vi "Positions Should Turn.vi"(8 "column":i32, 9 "row":i32, 10 "chess color":T2=1, 11 "chesses":T1=[[0, 1, 2, 0, 0, 0, 0], [0, 2, 1, 0, 0, 0, 0], [0, 0, 0, 2, 0, 0, 0], [0, 0, 0, 0, 0, 0, 0], [0, 0, 0, 0, 0, 0, 0]]) -> (1 "positons to turn":i32[][](array[numeric]), 3 "chesses new":T1=[[0, 1, 2, 0, 0, 0, 0], [0, 2, 1, 0, 0, 0, 0], [0, 0, 0, 2, 0, 0, 0], [0, 0, 0, 0, 0, 0, 0], [0, 0, 0, 0, 0, 0, 0]])   [LabVIEW 2018, in "Othello.xctl"]
doc: "本VI是为《我和LabVIEW》一书编写的示例。\n关于本书的介绍请参考网页：\nhttp://ruanqizhen.spaces.live.com/blog/cns!5852D4F797C53FB6!4310.entry"
uses:
  Othello.xctl
  Control/Pict Ring Chess.ctl
  Ability/Data.ctl
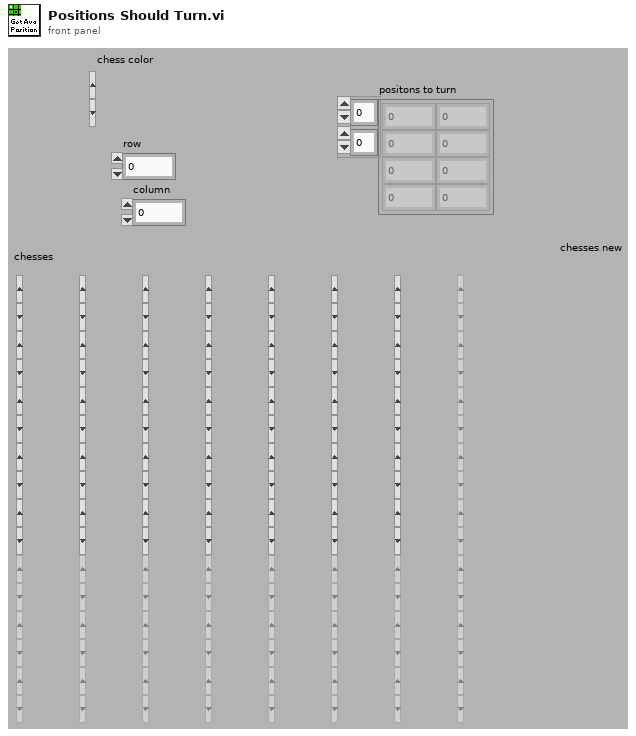
[diagram p1: front panel]
types:
  T1 = typedef "Othello.xctl/Data.ctl" = T2[][]
  T2 = typedef "Othello.xctl/Pict Ring Chess.ctl" = u16
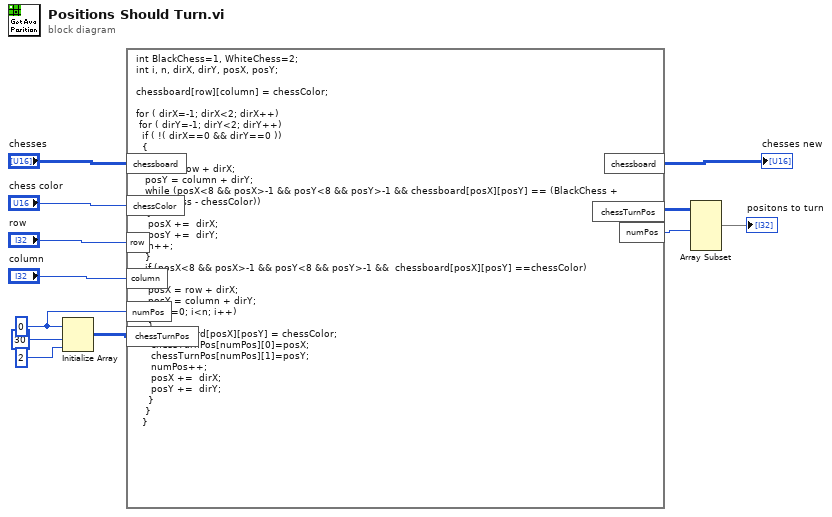
[diagram p0: block diagram]
diagram:
  w9 = 0 ("元素")
  n1 = Initialize Array(w9, 30 ("维数大小"), 2 ("维数大小")) -> (w11:i32[][])
  n2 = formula code="int BlackChess=1, WhiteChess=2;\nint i, n, dirX, dirY, posX, posY;\n\nchessboard[row][column] = chessColor;\n\nfor ( dirX=-1; dirX<2; dirX++)\n\tfor ( dirY=-1; dirY<2; dirY++)\n\t\tif ( !( dirX==0 && dirY==0 ))\n\t\t{\n\t\t\tn=0;\n\t\t\tposX = row + dirX;\n\t\t\tposY = column + dirY;\t\t\t\t\t\n\t\t\twhile (posX<8 && posX>-1 && posY<8 && posY>-1 && chessboard[posX][posY] == (BlackChess + WhiteChess - chessColor))\n\t\t\t{\n\t\t\t\tposX +=  dirX;\n\t\t\t\tposY +=  dirY;\n\t\t\t\tn++;\n\t\t\t}\n\t\t\tif (posX<8 && posX>-1 && posY<8 && posY>-1 &&  chessboard[posX][posY] ==chessColor)\n\t\t\t{\n\t\t\t\tposX = row + dirX;\n\t\t\t\tposY = column + dirY;\t\t\t\t\n\t\t\t\tfor (i=0; i<n; i++)\n\t\t\t\t{\n\t\t\t\t\tchessboard[posX][posY] = chessColor;\n\t\t\t\t\tchessTurnPos[numPos][0]=posX;\n\t\t\t\t\tchessTurnPos[numPos][1]=posY;\n\t\t\t\t\tnumPos++;\n\t\t\t\t\tposX +=  dirX;\n\t\t\t\t\tposY +=  dirY;\n\t\t\t\t}\n\t\t\t}\n\t\t}"("chessboard"="chesses", "chessTurnPos"=w11, "numPos"=w9, "chessColor"="chess color", "row"="row", "column"="column") -> ("chessTurnPos"=w7:i32[][], "numPos"=w6:i32, "chessboard"=→"chesses new":T1)
  n3 = Array Subset(array=w7, length (row)=w6) -> (→"positons to turn":i32[][])  [unwired: 3 in]
